vi "label_symmetry_v1.0.vi"() -> ()   [LabVIEW 2025]
doc: "Proof of concept/example VI for demonstration.\n\nMichael Panganiban\nSr. Hardware Test Engineer\nFresh Consulting, Inc."
uses:
  controls/home_navigation_btn.ctl
  controls/equipment_navigation_btn.ctl
  controls/settings_navigation_btn.ctl
  controls/test_plan_navigation_btn.ctl
  controls/queue_data.ctl
panel:
  in  "test_plan":T1
  in  "settings":T2
  in  "equipment":T3
  in  "home":T4
  in  "Tab":T5(tab)
  # "v1.0.0.1"
  # "HOME"
  # "EQUIPMENT"
  # "SETTINGS"
  # "HOME"
  # "TEST PLAN CREATION"
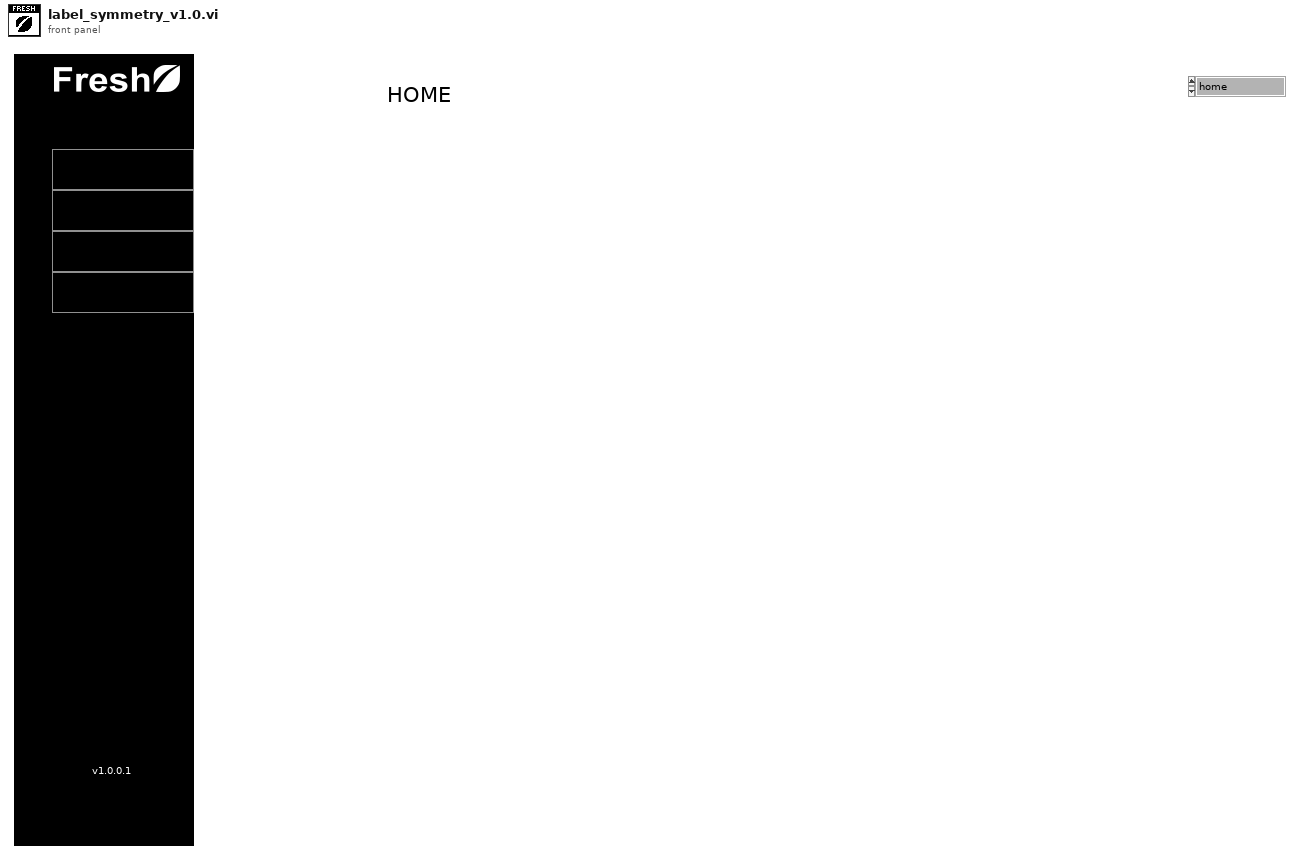
[diagram p1: front panel]
types:
  T1 = typedef "test_plan_navigation_btn.ctl" = bool
  T2 = typedef "settings_navigation_btn.ctl" = bool
  T3 = typedef "equipment_navigation_btn.ctl" = bool
  T4 = typedef "home_navigation_btn.ctl" = bool
  T5 = enum32{"home", "equipment", "settings", "test_plan"}
  T6 = typedef "queue_data.ctl" = cluster{"Action":string, "btn_ref":refnum<vi>}
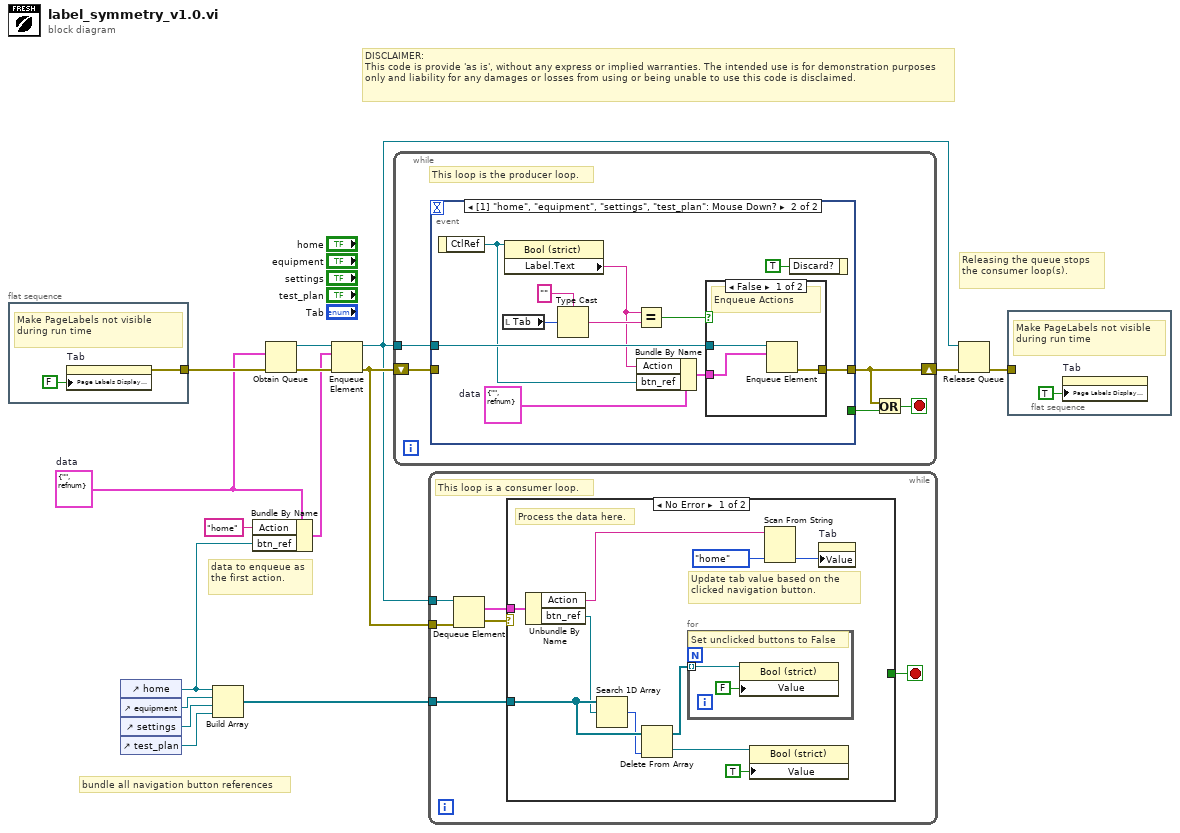
[diagram p0: block diagram]
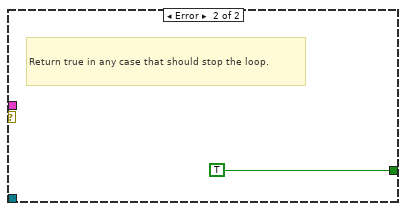
[diagram p2: hidden frame]
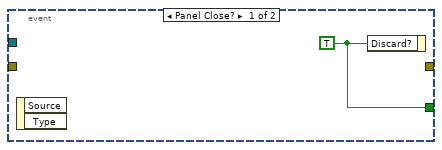
[diagram p3: hidden frame]
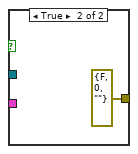
[diagram p4: hidden frame]
diagram:
  w6 = T6 {"Action"="", "btn_ref"=refnum}  # data
  # "data to enqueue as the first action."
  # "bundle all navigation button references"
  # "DISCLAIMER:\nThis code is provide 'as is', without any express or implied warranties. The intended use is for demonstration purposes only and liability for any damages or losses from using or being unable to use this code is disclaimed."
  # "Releasing the queue stops the consumer loop(s)."
  n1 = flat-sequence {
    tunnel: [w16] -> w14
    frame #0 {
      # "Make PageLabels not visible during run time"
      n2 = property on="Tab" class="TabCtl (strict)"("Page Labels Display Visible?"=FALSE) -> (error out=w16:errorcluster)  [unwired: 2 in, 1 out]
    }
  }
  n3 = control-ref of="home"() -> (w5:refnum<vi>)
  n4 = control-ref of="equipment"() -> (w12:refnum<vi>)
  n5 = control-ref of="settings"() -> (w11:refnum<vi>)
  n6 = control-ref of="test_plan"() -> (w10:refnum<vi>)
  n7 = Build Array(w5, w12, w11, w10) -> (w9:refnum<vi>[])
  n8 = Bundle By Name(cluster=w6, "Action"="home", "btn_ref"=w5) -> (w3:T6)
  n9 = Obtain Queue(element data type=w6, error in (no error)=w14) -> (queue out=w8:refnum<queue>, error out=w7:errorcluster)  [unwired: 3 in, 1 out]
  n10 = Enqueue Element(queue=w8, element=w3, error in (no error)=w7) -> (queue out=w1:refnum<queue>, error out=w2:errorcluster)  [unwired: 1 in, 1 out]
  n11 = while {
    shift-right: [w19] -> w15
    shift-left: w2 -> [w22]
    tunnel: w1 -> [w18]
    stop <- w20 stop-if-true
    # "This loop is the producer loop."
    n12 = event shown="[1] \"home\", \"equipment\", \"settings\", \"test_plan\": Mouse Down?" {
      selector: _ -> [_ _]
      dyn-events: _ -> [_ _]
      timeout: _ -> [_ _]
      tunnel: w18 -> [_ w31]
      tunnel: w22 -> [_ _]
      tunnel: [_ w32] -> w19
      tunnel: [w23 _] -> w21
      event Panel Close? {
        w23 = TRUE ("Discard?")
        n13 = event-data() -> ()  [unwired: 1 in, 2 out]
        n14 = event-data("Discard?"=w23) -> ()  [unwired: 1 in, 1 out]
      }
      event Mouse Down? {
        w33 = T6 {"Action"="", "btn_ref"=refnum}  # data
        n15 = event-data() -> ("CtlRef"=w30:refnum<vi>)  [unwired: 1 in]
        n16 = local read "Tab"() -> (w28:T5)
        n17 = property class="Bool (strict)"(reference=w30) -> ("Label.Text"=w25:string)  [unwired: 1 in, 2 out]
        n18 = Type Cast(type="", x=w28) -> (*(type *) &x=w26:string)
        n19 = Equal?(x=w25, y=w26) -> (x = y?=w24:bool)
        n20 = Bundle By Name(cluster=w33, "Action"=w25, "btn_ref"=w30) -> (w34:T6)
        n21 = case shown="False" w24 {
          tunnel: [w37 errorcluster {"status"=FALSE, "code"=0, "source"=""} ("error out")] -> w32
          tunnel: w31 -> [w36 _]
          tunnel: w34 -> [w35 _]
          frame False {
            # "Enqueue Actions"
            n22 = Enqueue Element(queue=w36, element=w35) -> (error out=w37:errorcluster)  [unwired: 2 in, 2 out]
          }
          frame True {
          }
        }
        n23 = event-data("Discard?"=TRUE) -> ()  [unwired: 1 in, 1 out]
      }
    }
    n24 = Or(x=w19, y=w21) -> (x .or. y?=w20:bool)
  }
  n25 = while {
    tunnel: w1 -> [w44]
    tunnel: w9 -> [w40]
    tunnel: w2 -> [w39]
    stop <- w41 stop-if-true
    # "This loop is a consumer loop."
    n26 = Dequeue Element(queue=w44, error in (no error)=w39) -> (element=w42:T6, error out=w43:errorcluster)  [unwired: 1 in, 2 out]
    n27 = case shown="No Error" w43 {
      tunnel: w42 -> [w54 _]
      tunnel: [_ TRUE] -> w41
      tunnel: w40 -> [w53 _]
      frame No Error {
        # "Update tab value based on the clicked navigation button."
        # "Process the data here."
        n28 = Unbundle By Name(w54) -> ("Action"=w47:string, "btn_ref"=w48:refnum<vi>)
        n29 = Search 1D Array(1D array=w53, element=w48) -> (index of element=w52:i32)  [unwired: 1 in]
        n30 = Delete From Array "Delete From Array"(array=w53, index=w52) -> (deleted portion=w51:refnum<vi>, array with subset deleted=w49:refnum<vi>[])  [unwired: 1 in]
        n31 = for {
          tunnel: w49 -> [w55] mode=indexing
          # "Set unclicked buttons to False"
          n32 = property class="Bool (strict)"(reference=w55, "Value"=T4 FALSE) -> ()  [unwired: 1 in, 2 out]
        }
        n33 = property class="Bool (strict)"(reference=w51, "Value"=T4 TRUE) -> ()  [unwired: 1 in, 2 out]
        n34 = Scan From String(input string=w47, default 1=T5."home" ("Tab Control")) -> (output 1=w45:T5)  [unwired: 3 in, 3 out]
        n35 = property on="Tab" class="TabCtl (strict)"("Value"=w45) -> ()  [unwired: 2 in, 2 out]
      }
      frame Error {
        # "Return true in any case that should stop the loop."
      }
    }
  }
  n36 = Release Queue(queue=w1, error in (no error)=w15) -> (error out=w13:errorcluster)  [unwired: 1 in, 2 out]
  n37 = flat-sequence {
    tunnel: w13 -> [_]
    frame #0 {
      # "Make PageLabels not visible during run time"
      n38 = property on="Tab" class="TabCtl (strict)"("Page Labels Display Visible?"=TRUE) -> ()  [unwired: 2 in, 2 out]
    }
  }
